vi "Token SInk.vi"(2 "token 1":T1, 3 "token 2":T1) -> (7 "token out":T1)   [LabVIEW 2023]
uses:
  <extravilib>/ChannelInstances/One Element Stream-bool/)Channel.ctl
  <extravilib>/ChannelInstances/One Element Stream-bool/Read With Abort.vi
  <extravilib>/ChannelInstances/One Element Stream-bool/Write With Abort.vi
  <extravilib>/ChannelInstances/One Element Stream-bool/EndpointRead.vi
  <extravilib>/ChannelInstances/One Element Stream-bool/Endpoint.vi
  <extravilib>/ChannelInstances/One Element Stream-bool.lvlib
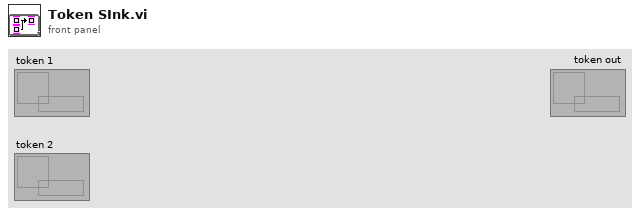
[diagram p1: front panel]
types:
  T1 = typedef "One Element Stream-bool.lvlib/)Channel.ctl" = refnum<queue>
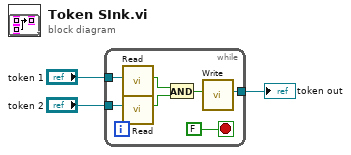
[diagram p0: block diagram]
diagram:
  n1 = while {
    tunnel: "token 1" -> [w10]
    tunnel: "token 2" -> [w9]
    tunnel: [w4] -> w1
    stop <- FALSE stop-if-true
    n2 = call <extravilib>:"Read.vi"("channel"=w10) -> ("element"=w7:bool)  [unwired: 7 in, 3 out]
    n3 = call <extravilib>:"Read.vi"("channel"=w9) -> ("element"=w6:bool)  [unwired: 7 in, 3 out]
    n4 = And(x=w7, y=w6) -> (x .and. y?=w5:bool)
    n5 = call <extravilib>:"Write.vi"("element"=w5) -> ("channel"=w4:T1)  [unwired: 9 in, 1 out]
  }
  "token out" <- w1
